vi "Maximize.vi"(4 "PlotPane":refnum<vi>, 6 "Front Panel":refnum<vi>, 8 "error in (no error)":errorcluster, 9 "owning subpanel":refnum<vi>, 10 "maximize button data":T1, 11 "Loop data in":T2 {"PanelMap"."Data"."Plot Bounds (%)"."Bottom (%)" format="%.2f"; "PanelMap"."Data"."Plot Bounds (%)"."Top (%)" format="%.2f"; "PanelMap"."Data"."Plot Bounds (%)"."Right (%)" format="%.2f"; "PanelMap"."Data"."Plot Bounds (%)"."Left (%)" format="%.2f"}) -> (0 "error out":errorcluster, 3 "Loop data out":T2 {"PanelMap"."Data"."Plot Bounds (%)"."Bottom (%)" format="%.2f"; "PanelMap"."Data"."Plot Bounds (%)"."Top (%)" format="%.2f"; "PanelMap"."Data"."Plot Bounds (%)"."Right (%)" format="%.2f"; "PanelMap"."Data"."Plot Bounds (%)"."Left (%)" format="%.2f"})   [LabVIEW 2021, in "MultiStokePlot.lvlib" / "MultiPlotPanel.lvclass"]
uses:
  MultiPlotPanel.lvclass
  SubVIs/Loop Data.ctl
  <vilib>/IlluminatedG/IG OOPanel/OOPanel/Manager/Manager.lvclass
  SubVIs/Panel Map.ctl
  SubVIs/Panel Map Data.ctl
  <userlib>/bjustice/RocketPlot/Classes/RocketPlotPanel/RocketPlotPanel.lvclass
  C:/Program Files/National Instruments/LabVIEW 2021/vi.lib/IlluminatedG/IG OOPanel/OOPanel/Panel/Panel.lvclass
  SubVIs/Window Position.ctl
  <vilib>/IlluminatedG/IG OOPanel/OOPanel/Panel/Panel Events.ctl
  <vilib>/IlluminatedG/IG OOPanel/OOPanel/Panel/Visbility Event Data.ctl
  <vilib>/IlluminatedG/IG OOPanel/OOPanel/Visibility State.ctl
  <vilib>/IlluminatedG/IG OOPanel/OOPanel/Close Reason.ctl
  <userlib>/bjustice/RocketPlot/Classes/RocketPlotHandle/SubVIs/callback maximize data.ctl
  <vilib>/Utility/miscctls.llb/LVMapReplaceAction.ctl
  <vilib>/IlluminatedG/IG OOPanel/OOPanel/Panel/Panel.lvclass
  <userlib>/bjustice/RocketPlot/Classes/RocketPlotHandle/RocketPlotHandle.lvclass
  <vilib>/IlluminatedG/IG OOPanel/OOPanel/OOPanel.lvlib
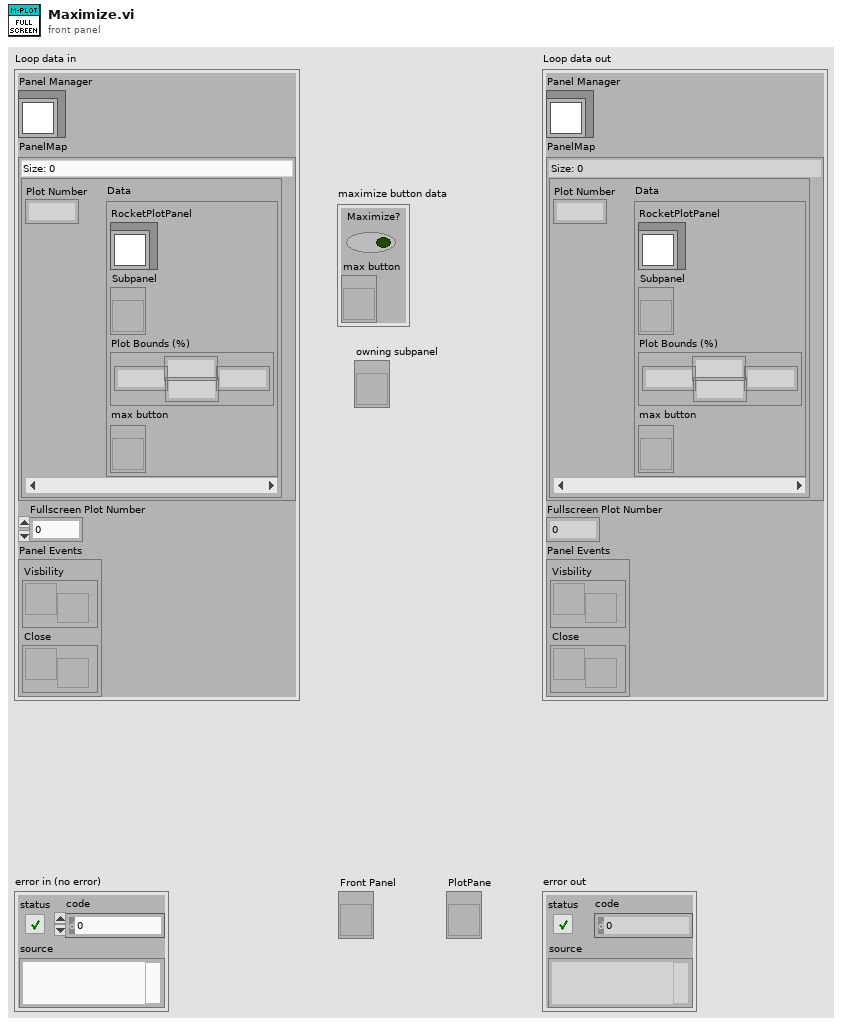
[diagram p1: front panel]
types:
  T1 = typedef "RocketPlotHandle.lvclass/callback maximize data.ctl" = cluster{"Maximize?":bool, "max button":refnum<vi>}
  T2 = typedef "MultiStokePlot.lvlib/MultiPlotPanel.lvclass/Loop Data.ctl" = cluster{"Panel Manager":refnum<class "Manager.lvclass">, "PanelMap":T3, "Fullscreen Plot Number":i32, "Panel Events":T6}
  T3 = typedef "MultiStokePlot.lvlib/MultiPlotPanel.lvclass/Panel Map.ctl" = map{i32, T4}
  T4 = typedef "MultiStokePlot.lvlib/MultiPlotPanel.lvclass/Panel Map Data.ctl" = cluster{"RocketPlotPanel":refnum<class "RocketPlotPanel.lvclass">, "Subpanel":refnum<vi>, "Plot Bounds (%)":T5, "max button":refnum<vi>}
  T5 = typedef "MultiStokePlot.lvlib/MultiPlotPanel.lvclass/Window Position.ctl" = cluster{"Left (%)":dbl, "Top (%)":dbl, "Right (%)":dbl, "Bottom (%)":dbl}
  T6 = typedef "OOPanel.lvlib/Panel.lvclass/Panel Events.ctl" = cluster{"Visbility":refnum<user-event>, "Close":refnum<user-event>}
  T7 = typedef "LVMapReplaceAction.ctl" = enum32{"Modify Entry only if found", "Add or Modify Entry", "Delete Entry"}
  T8 = typedef "LVRectTypeDef.ctl" = cluster{"Left":i16, "Top":i16, "Right":i16, "Bottom":i16}
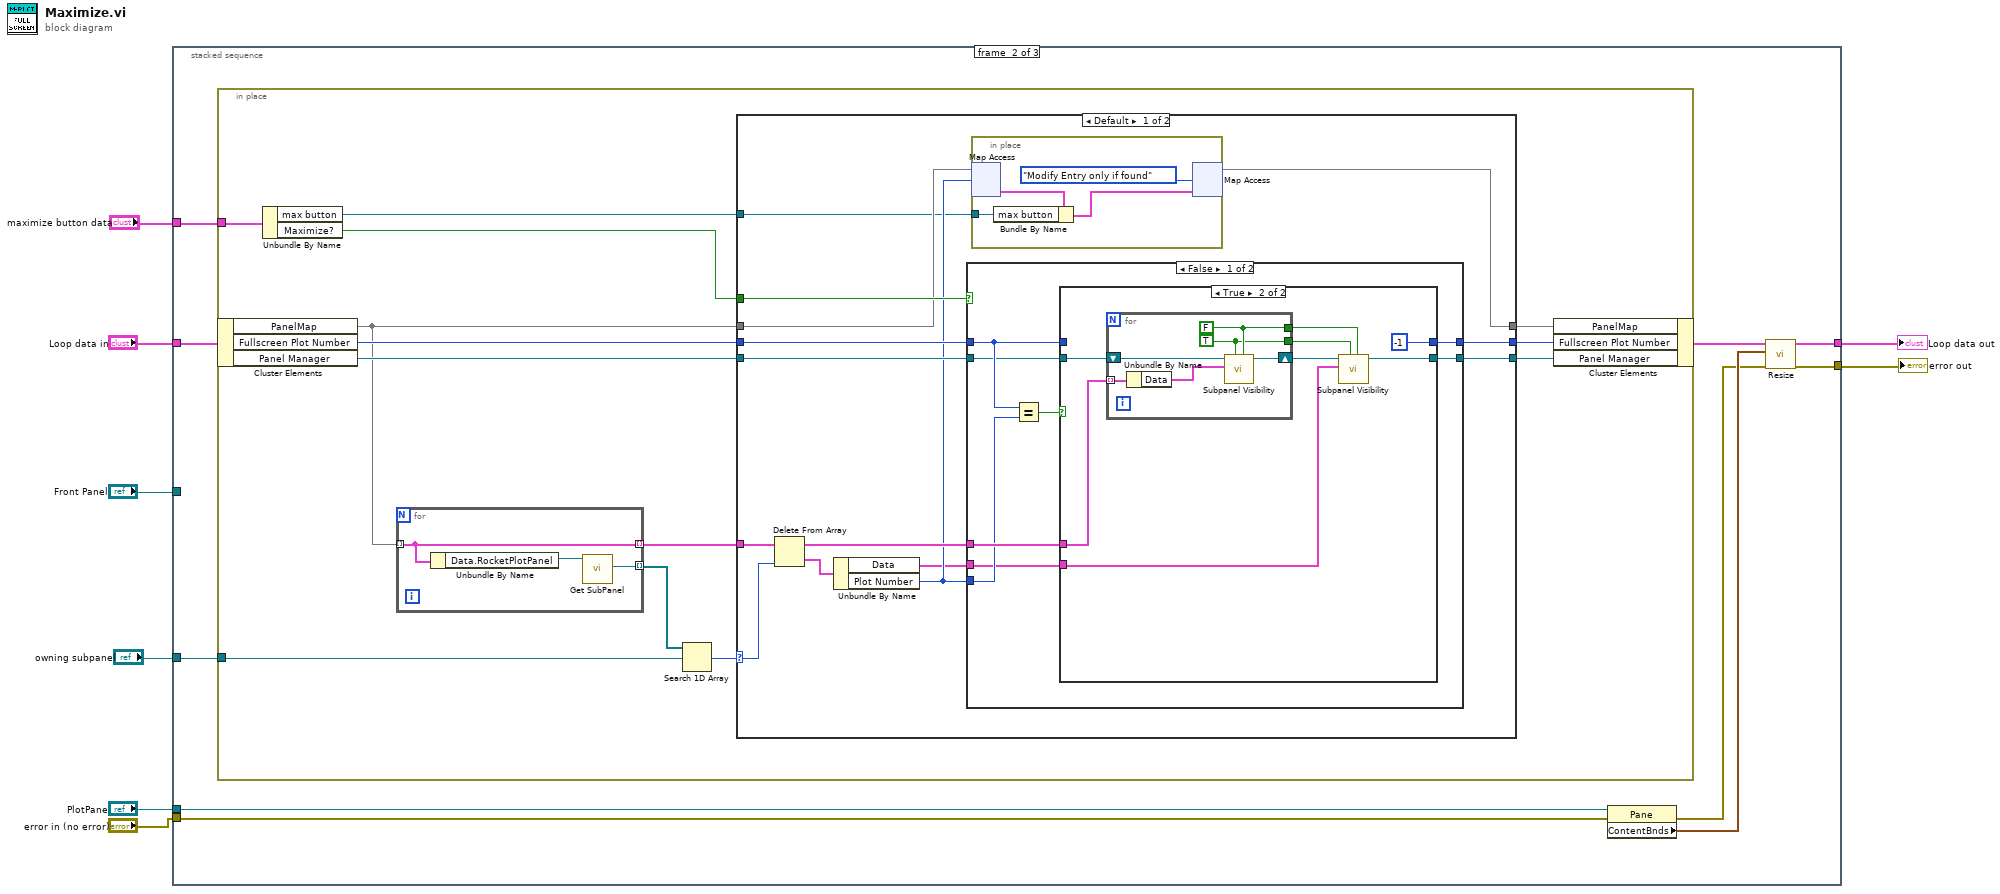
[diagram p0: block diagram]
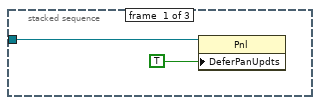
[diagram p2: hidden frame]
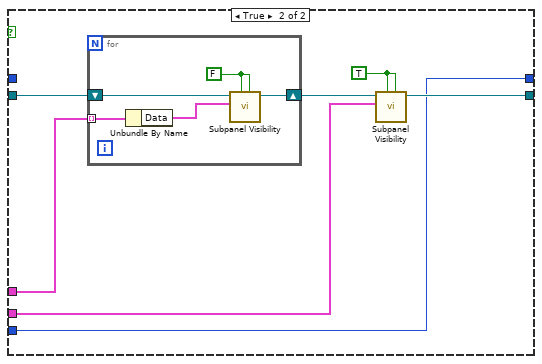
[diagram p4: hidden frame]
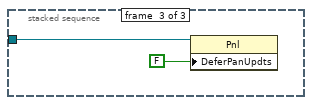
[diagram p6: hidden frame]
diagram:
  n1 = stacked-sequence {
    tunnel: "Loop data in" -> [_ w20 _]
    tunnel: "owning subpanel" -> [_ w19 _]
    tunnel: "PlotPane" -> [_ w17 _]
    tunnel: [_ w15 _] -> w6
    tunnel: "error in (no error)" -> [_ w14 _]
    tunnel: [_ w12 _] -> w4
    tunnel: "Front Panel" -> [w10 _ w94]
    tunnel: "maximize button data" -> [_ w11 _]
    frame #0 {
      n2 = property class="Pnl"(reference=w10, "DeferPanUpdts"=TRUE ("Defer Panel Updates")) -> ()  [unwired: 1 in, 2 out]
    }
    frame #1 {
      n3 = in-place {
        in-place-border: w19 -> [w21]
        in-place-border: w11 -> [w22]
        n4 = in-place-cluster #1(w20) -> ("PanelMap"=w26:T3, "Fullscreen Plot Number"=w30:i32, "Panel Manager"=w28:refnum<class "Manager.lvclass">)
        n5 = Unbundle By Name(w22) -> ("max button"=w24:refnum<vi>, "Maximize?"=w23:bool)
        n6 = for {
          tunnel: w26 -> [w36] mode=indexing
          tunnel: [w34] -> w33 mode=indexing
          tunnel: [w36] -> w29 mode=indexing
          n7 = Unbundle By Name(w36) -> ("Data.RocketPlotPanel"=w35:refnum<class "RocketPlotPanel.lvclass">)
          n8 = call <vilib>:"Get SubPanel.vi"("Panel in"=w35) -> ("SubPanel"=w34:refnum<vi>)  [unwired: 8 in, 2 out]
        }
        n9 = Search 1D Array(1D array=w33, element=w21) -> (index of element=w32:i32)  [unwired: 1 in]
        n10 = case shown="Default" w32 {
          selector: w32 -> [w42 _]
          tunnel: [w49 w93] -> w31
          tunnel: w30 -> [w48 w93]
          tunnel: w29 -> [w47 _]
          tunnel: w23 -> [w50 _]
          tunnel: w28 -> [w45 w92]
          tunnel: [w44 w92] -> w27
          tunnel: w26 -> [w43 w91]
          tunnel: w24 -> [w39 _]
          tunnel: [w38 w91] -> w25
          frame Default {
            n11 = Delete From Array(array=w47, index=w42) -> (deleted portion=w41:cluster{"Plot Number":i32, "Data":T4}, array with subset deleted=w46:cluster{"Plot Number":i32, "Data":T4}[])  [unwired: 1 in]
            n12 = Unbundle By Name(w41) -> ("Data"=w37:T4, "Plot Number"=w40:i32)
            n13 = case shown="False" w50 {
              tunnel: [w61 w81] -> w49
              tunnel: w48 -> [w60 _]
              tunnel: w46 -> [w59 w85]
              tunnel: w45 -> [w58 w84]
              tunnel: [w57 w82] -> w44
              tunnel: w40 -> [w56 w81]
              tunnel: w37 -> [w55 w80]
              frame False {
                n14 = Equal?(x=w60, y=w56) -> (x = y?=w62:bool)
                n15 = case shown="True" w62 {
                  tunnel: [w64 -1 ("Fullscreen Plot Number")] -> w61
                  tunnel: w60 -> [w64 _]
                  tunnel: w59 -> [_ w69]
                  tunnel: w58 -> [w63 w70]
                  tunnel: [w63 w68] -> w57
                  tunnel: w55 -> [_ w65]
                  frame False {
                  }
                  frame True {
                    n16 = for {
                      tunnel: w69 -> [w78] mode=indexing
                      shift-right: [w76] -> w71
                      shift-left: w70 -> [w77]
                      tunnel: [w74] -> w67
                      tunnel: [w73] -> w66
                      w74 = FALSE ("Maximized?")
                      w73 = TRUE ("Visible")
                      n17 = Unbundle By Name(w78) -> ("Data"=w75:T4)
                      n18 = call "Subpanel Visibility.vi"("Maximized?"=w74, "Visible"=w73, "Panel"=w75, "Manager in"=w77) -> ("Manager out"=w76:refnum<class "Manager.lvclass">)  [unwired: 6 in, 1 out]
                    }
                    n19 = call "Subpanel Visibility.vi"("Maximized?"=w67, "Visible"=w66, "Panel"=w65, "Manager in"=w71) -> ("Manager out"=w68:refnum<class "Manager.lvclass">)  [unwired: 6 in, 1 out]
                  }
                }
              }
              frame True {
                w79 = TRUE ("Visible")
                n20 = for {
                  tunnel: w85 -> [w88] mode=indexing
                  shift-right: [w89] -> w83
                  shift-left: w84 -> [w90]
                  w86 = FALSE ("Visible")
                  n21 = Unbundle By Name(w88) -> ("Data"=w87:T4)
                  n22 = call "Subpanel Visibility.vi"("Maximized?"=w86, "Visible"=w86, "Panel"=w87, "Manager in"=w90) -> ("Manager out"=w89:refnum<class "Manager.lvclass">)  [unwired: 6 in, 1 out]
                }
                n23 = call "Subpanel Visibility.vi"("Maximized?"=w79, "Visible"=w79, "Panel"=w80, "Manager in"=w83) -> ("Manager out"=w82:refnum<class "Manager.lvclass">)  [unwired: 6 in, 1 out]
              }
            }
            n24 = in-place {
              in-place-border: w39 -> [w51]
              n25 = in-place-map #2(w43, w40) -> (w54:T4)  [unwired: 1 in, 1 out]
              n26 = Bundle By Name(cluster=w54, "max button"=w51) -> (w53:T4)
              n27 = in-place-map #2(w53, LVMapReplaceAction."Modify Entry only if found" ("action")) -> (w38:T3)  [unwired: 2 out]
            }
          }
          frame -1 {
          }
        }
        n28 = in-place-cluster #1("PanelMap"=w25, "Fullscreen Plot Number"=w31, "Panel Manager"=w27) -> (w18:T2)
      }
      n29 = property on="Property Node" class="Pane"(reference=w17, error in=w14) -> (error out=w13:errorcluster, "ContentBnds"=w16:T8)  [unwired: 1 out]
      n30 = call "Resize.vi"("error in (no error)"=w13, "Pane.Content Area Rect"=w16, "Loop data in"=w18) -> ("error out"=w12:errorcluster, "Loop data out"=w15:T2)  [unwired: 7 in]
    }
    frame #2 {
      n31 = property class="Pnl"(reference=w94, "DeferPanUpdts"=FALSE ("Defer Panel Updates")) -> ()  [unwired: 1 in, 2 out]
    }
  }
  "Loop data out" <- w6
  "error out" <- w4
